vi "TemperatureDemo.vi"() -> ()   [LabVIEW 2015]
panel:
  in  "Measurement Function (10: Voltage DC)":i32(ring)=10 items=["Continuity", "Current AC", "Current DC", "Diode", "Frequency", "Resistance 4-wire", "Period", "Resistance 2-wire", "Temperature", "Voltage AC", "Voltage DC", "Voltage DC Ratio"]
  out "Measurement":dbl
  in  "VISA resource name":refnum<visa-resource-name>="TCPIP0::K-34461A-22329.local::inst0::INSTR"
  out "error out":errorcluster
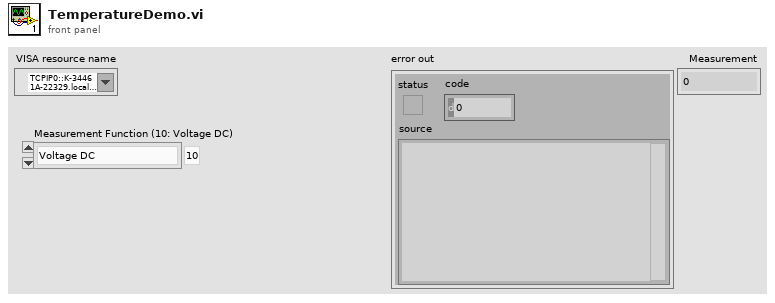
[diagram p1: front panel]
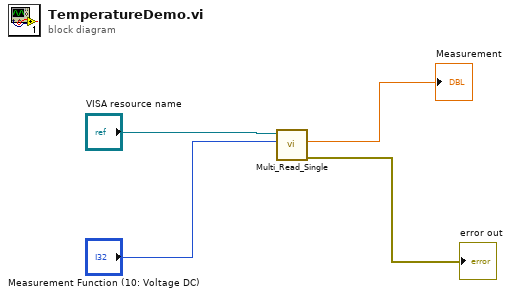
[diagram p0: block diagram]
diagram:
  n1 = call "Multi_Read_Single.vi"("Measurement Function (10: Voltage DC)"="Measurement Function (10: Voltage DC)", "VISA resource name"="VISA resource name") -> ("error out"=→"error out":errorcluster, "Measurement"=→"Measurement":dbl)  [unwired: 8 in]
